vi "GetFunctionConfig.vi"(8 "error in (no error)":errorcluster, 11 "ArbitraryFunction In":refnum<class "ArbitraryFunction.lvclass">) -> (0 "error out":errorcluster, 2 "FunctionConfig":variant, 3 "ArbitraryFunction Out":refnum<class "ArbitraryFunction.lvclass">)   [LabVIEW 2018, in "Functions.lvlib" / "ArbitraryFunction.lvclass"]
uses:
  ArbitraryFunction.lvclass
  ArbitraryFunction.lvclass/ArbitraryFunction.ctl
  TypeDefs/Arbs.ctl
  Accessors/Read SampleRate.vi
  Accessors/Read Arbs.vi
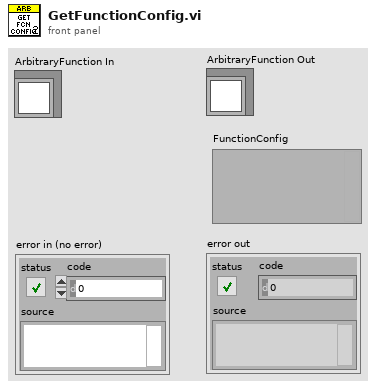
[diagram p1: front panel]
types:
  T1 = cluster{"Arbs":cluster{"Handle":string, "Size":i32, "Gain":dbl, "Offset":dbl}[], "SampleRate":dbl, "SettlingTime":dbl, "T0":dbl}
  T2 = typedef "Functions.lvlib/ArbitraryFunction.lvclass/Arbitrary.ctl" = cluster{"Handle":string, "Size":i32, "Gain":dbl, "Offset":dbl, "Waveform":waveform(dbl)}
  T3 = typedef "Functions.lvlib/ArbitraryFunction.lvclass/Arbs.ctl" = cluster{"Handle":string, "Size":i32, "Gain":dbl, "Offset":dbl}
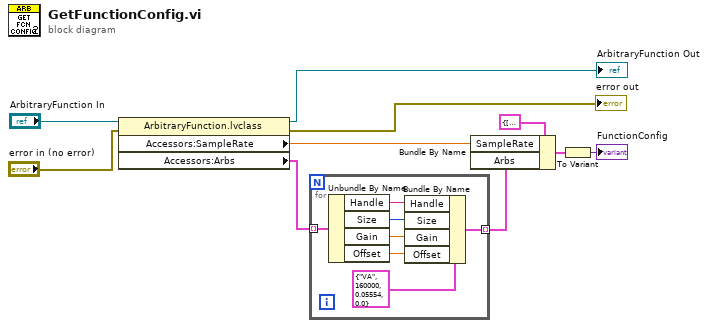
[diagram p0: block diagram]
diagram:
  n1 = property class="ArbitraryFunction.lvclass"(reference="ArbitraryFunction In", error in="error in (no error)") -> (reference out=→"ArbitraryFunction Out":refnum<class "ArbitraryFunction.lvclass">, error out=→"error out":errorcluster, "Accessors:SampleRate"=w6:dbl, "Accessors:Arbs"=w8:T2[])
  n2 = for {
    tunnel: w8 -> [w17] mode=indexing
    tunnel: [w11] -> w5 mode=indexing
    n3 = Unbundle By Name(w17) -> ("Handle"=w15:string, "Size"=w14:i32, "Gain"=w13:dbl, "Offset"=w12:dbl)
    n4 = Bundle By Name(cluster=T3 {"Handle"="VA", "Size"=160000, "Gain"=0.05554, "Offset"=0.0} ("Arbs"), "Handle"=w15, "Size"=w14, "Gain"=w13, "Offset"=w12) -> (w11:T3)
  }
  n5 = Bundle By Name(cluster=T1 {"Arbs"=[], "SampleRate"=0.0, "SettlingTime"=0.0, "T0"=0.0} ("FunctionConfig"), "SampleRate"=w6, "Arbs"=w5) -> (w4:T1)
  n6 = To Variant(anything=w4) -> (Variant=→"FunctionConfig":variant)
